vi "cmd_vi_01.vi"() -> ()   [LabVIEW 2010]
doc: "Demonstrates how to set up a basic TCP connection, send data to the specified port once a connection has been established, and terminate the connection once the data has been sent. This VI is designed to stop if the TCP connection is terminated.\n\nThe data sent in this example is an array consisting of one of three user selectable waveforms.\n\n<B>Note:</B> Requires the Simple Data Client.vi located in the same library as this VI."
panel:
  out "Out":string
  out "error out":errorcluster
  out "data out":string
  in  "stop":bool
  in  "Port":u16=5010 min=1025 step=1
  # "Instructions:\n1. Open the Simple Data Client.vi.\n2. Run this VI first.\n3. Run the Simple Data Client.vi second.\n4. Adjust the Function and # of Points controls to see the plot on the front panel of the Simple Data Client.vi change.\n\nNote:  This VI will time out after 60 seconds if no connection is detected."
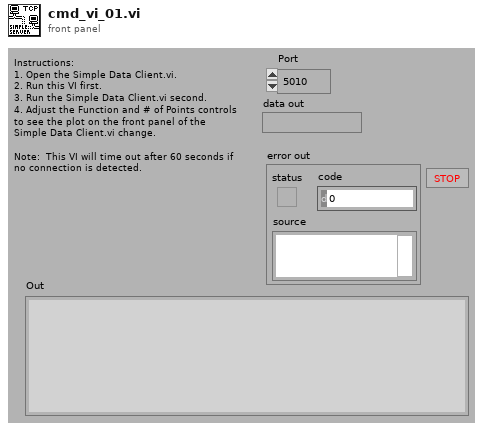
[diagram p1: front panel]
types:
  T1 = enum16{"Standard", "Buffered", "CRLF", "Immediate"}
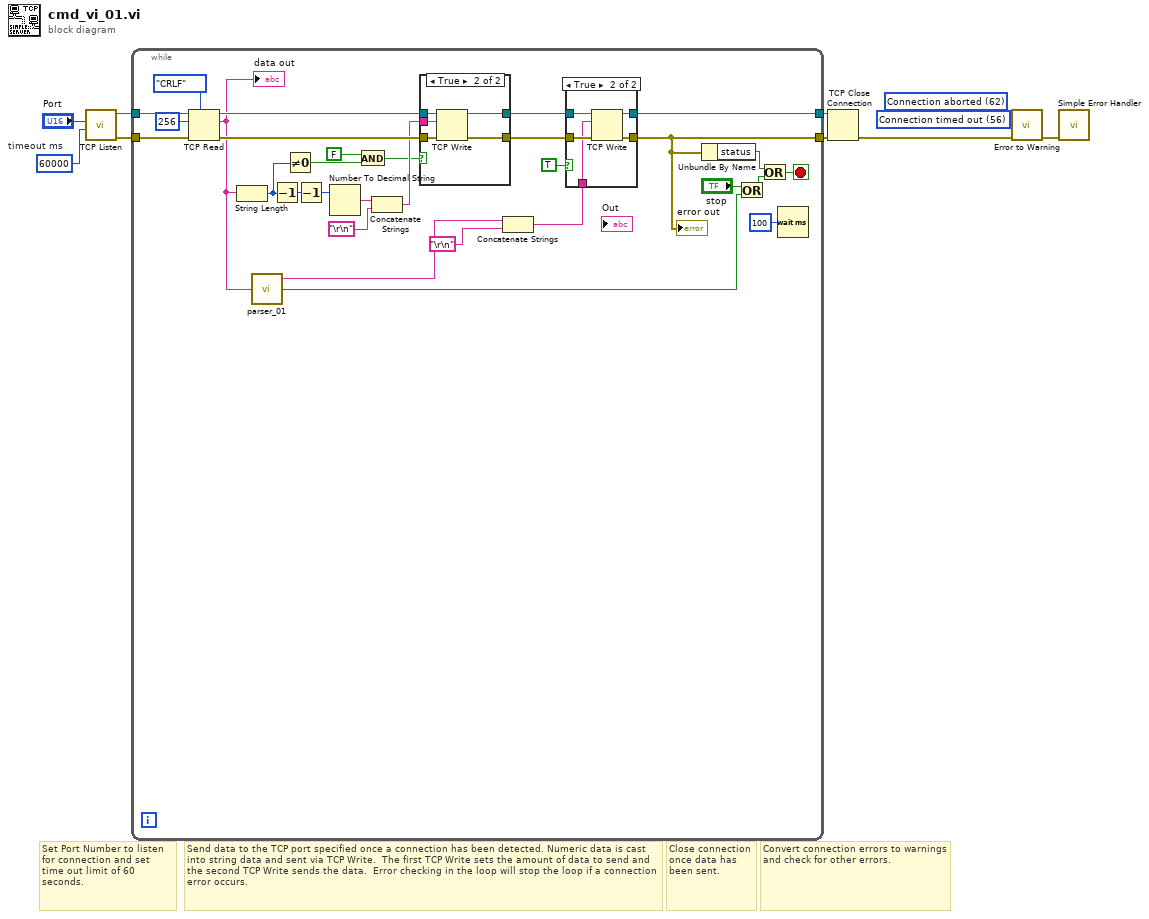
[diagram p0: block diagram]
diagram:
  w1 = 60000  # timeout ms
  w6 = 56 items=["No Error", "Argument Error", "Memory Full", "Out of Zone", "End of File", "File Already Open", "Generic File IO Error", "File Not Found", "File Permission Error", "Disk Full", "Duplicate Path", "Too Many Files Open", "Not Enabled", "Resource File Not Found", "Cannot Add Resource", "Resource Not Found", "Image Not Found", "Image Memory Error", "Pen Does Not Exist", "Config Bad Type", "Config Token Not Found", "Config Parse Error", "Config Memory Error", "Bad External Code Format", "Bad External Code Offset", "External Code Not Present", "Null Window", "Destroy Window Mixup", "Null Menu", "Print Aborted", "Bad Print Record", "Print Driver Error", "Windows Error During Print", "Memory Error During Print", "Print Dialog Error", "Generic Print Error", "Invalid Device Refnum", "Device Not Found", "Device Parameter Error", "Device Unit Error", "Can't Open Device", "Device Call Aborted", "Generic Error", "Cancelled By User", "Object ID Too Low", "Object ID Too High", "Object Not In Heap", "Unknown Heap", "Bad DefProc ID", "DefProc Not In Table", "Message Out Of Range", "Null Method", "Unknown Message", "Manager Call Not Supported", "Bad address", "Connection In progress", "Connection timed out", "Connection is already in progress", "Network attribute not supported", "Network error", "Address in use", "System out of memory", "Connection aborted", "Connection refused", "Connection is not connected", "Connection is already connected", "Connection closed", "Initialize error (interapplication manager)", "Bad occurrence", "Wait on unbound occurrence handler", "Occurrence queue overflow", "Bad path", "Semaphore not signaled", "Unrecognized type (interapplication manager)"] ("2nd Error to Convert")
  w7 = 62 items=["No Error", "Argument Error", "Memory Full", "Out of Zone", "End of File", "File Already Open", "Generic File IO Error", "File Not Found", "File Permission Error", "Disk Full", "Duplicate Path", "Too Many Files Open", "Not Enabled", "Resource File Not Found", "Cannot Add Resource", "Resource Not Found", "Image Not Found", "Image Memory Error", "Pen Does Not Exist", "Config Bad Type", "Config Token Not Found", "Config Parse Error", "Config Memory Error", "Bad External Code Format", "Bad External Code Offset", "External Code Not Present", "Null Window", "Destroy Window Mixup", "Null Menu", "Print Aborted", "Bad Print Record", "Print Driver Error", "Windows Error During Print", "Memory Error During Print", "Print Dialog Error", "Generic Print Error", "Invalid Device Refnum", "Device Not Found", "Device Parameter Error", "Device Unit Error", "Can't Open Device", "Device Call Aborted", "Generic Error", "Cancelled By User", "Object ID Too Low", "Object ID Too High", "Object Not In Heap", "Unknown Heap", "Bad DefProc ID", "DefProc Not In Table", "Message Out Of Range", "Null Method", "Unknown Message", "Manager Call Not Supported", "Bad address", "Connection In progress", "Connection timed out", "Connection is already in progress", "Network attribute not supported", "Network error", "Address in use", "System out of memory", "Connection aborted", "Connection refused", "Connection is not connected", "Connection is already connected", "Connection closed", "Initialize error (interapplication manager)", "Bad occurrence", "Wait on unbound occurrence handler", "Occurrence queue overflow", "Bad path", "Semaphore not signaled", "Unrecognized type (interapplication manager)"] ("1st Error to Convert")
  # "Convert connection errors to warnings and check for other errors."
  # "Close connection once data has been sent."
  # "Send data to the TCP port specified once a connection has been detected. Numeric data is cast into string data and sent via TCP Write.  The first TCP Write sets the amount of data to send and the second TCP Write sends the data.  Error checking in the loop will stop the loop if a connection error occurs."
  # "Set Port Number to listen for connection and set time out limit of 60 seconds."
  n1 = call <vilib>:"TCP Listen.vi"("timeout ms (wait forever: -1)"=w1, "port"="Port") -> ("error out"=w2:errorcluster, "connection ID"=w4:refnum<k5>)  [unwired: 6 in, 2 out]
  n2 = while {
    tunnel: [w21] -> w3
    tunnel: [w22] -> w5
    tunnel: w4 -> [w39]
    tunnel: w2 -> [w35]
    stop <- w37 stop-if-true
    n3 = TCP Read(connection ID=w39, bytes to read=256, 7:T1."CRLF" ("mode (standard)")) -> (connection ID out=w32:refnum<k5>, data out=w20:string)  [unwired: 2 in, 1 out]
    "data out" <- w20
    n4 = String Length(string=w20) -> (length=w30:i32)
    n5 = call "parser_01.vi"("data in"=w20) -> ("Exit"=w26:bool, "Answer"=w12:string)  [unwired: 3 in]
    n6 = Decrement(x=w30) -> (x-1=w23:i32)
    n7 = Not Equal To 0?(x=w30) -> (x != 0?=w17:bool)
    n8 = Decrement(x=w23) -> (x-1=w19:i32)
    n9 = Number To Decimal String(number=w19) -> (decimal integer string=w31:string)  [unwired: 1 in]
    n10 = And(x=FALSE, y=w17) -> (x .and. y?=w18:bool)
    n11 = Concatenate Strings(w31, "\r\n") -> (w25:string)
    n12 = case shown="True" w18 {
      tunnel: w35 -> [w47 w53]
      tunnel: [w47 w52] -> w15
      tunnel: [w48 w51] -> w33
      tunnel: w32 -> [w48 w50]
      tunnel: w25 -> [_ w49]
      frame False {
      }
      frame True {
        n13 = TCP Write(connection ID=w50, data in=w49, error in (no error)=w53) -> (connection ID out=w51:refnum<k5>, error out=w52:errorcluster)  [unwired: 1 in, 1 out]
      }
    }
    n14 = Concatenate Strings(w12, "\r\n") -> (w11:string)
    n15 = case shown="True" TRUE {
      tunnel: w33 -> [w41 w46]
      tunnel: [w41 w45] -> w22
      tunnel: [w40 w44] -> w21
      tunnel: w15 -> [w40 w43]
      tunnel: w11 -> [_ w42]
      frame False {
      }
      frame True {
        n16 = TCP Write(connection ID=w46, data in=w42, error in (no error)=w43) -> (connection ID out=w45:refnum<k5>, error out=w44:errorcluster)  [unwired: 1 in, 1 out]
      }
    }
    "error out" <- w21
    n17 = Unbundle By Name(w21) -> ("status"=w36:bool)
    n18 = Or(x="stop", y=w26) -> (x .or. y?=w27:bool)
    n19 = Or(x=w36, y=w27) -> (x .or. y?=w37:bool)
    n20 = Wait (ms)(milliseconds to wait=u32 100) -> ()  [unwired: 1 out]
  }
  n21 = TCP Close Connection(connection ID=w5, error in (no error)=w3) -> (error out=w9:errorcluster)  [unwired: 1 in, 1 out]
  n22 = call <vilib>:"Error to Warning.vi"("1st Error to Convert"=w7, "2nd Error to Convert"=w6, "error in"=w9) -> ("warning out"=w8:errorcluster)  [unwired: 12 in]
  n23 = call <vilib>:"Simple Error Handler.vi"("error in (no error)"=w8) -> ()  [unwired: 4 in, 5 out]
